vi "POC State.vi"(8 "error in (no error)":errorcluster, 11 "Node Ptr":T1 format="%.0x") -> (0 "error out":errorcluster)   [LabVIEW 2020, in "FlexRay Custom Device System Explorer.lvlib"]
uses:
  FlexRay Custom Device System Explorer.lvlib
  <vilib>/NI VeriStand/Custom Device API/Custom Device Item Ref.ctl
  <vilib>/NI VeriStand/Custom Device API/Custom Device API.lvlib
panel:
  in  "Header":cluster{"Section Name":string}={"Section Name"="Custom Device Item Settings"}
  in  "Description":string="POC State:\n0: Default Config\n1: Ready\n2: Normal Active\n3: Normal Passive\n4: Halt\n15: Config"
  in  "Name":string
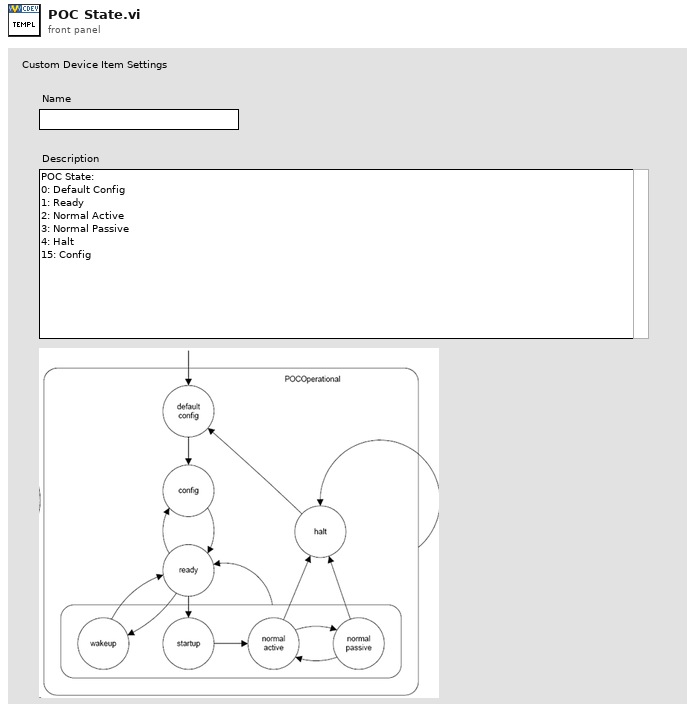
[diagram p1: front panel]
types:
  T1 = typedef "Custom Device API.lvlib/Custom Device Item Ref.ctl" = u64
  T2 = typedef "Custom Device API.lvlib/Custom Device Item Info.ctl" = cluster{"Name":string, "Is Channel":bool, "GUID":string, "Is Waveform":bool}
  T3 = typedef "Custom Device API.lvlib/Custom Device Commands.ctl" = enum16{"Default", "Item renamed", "Shutdown", "Dynamic button pressed"}
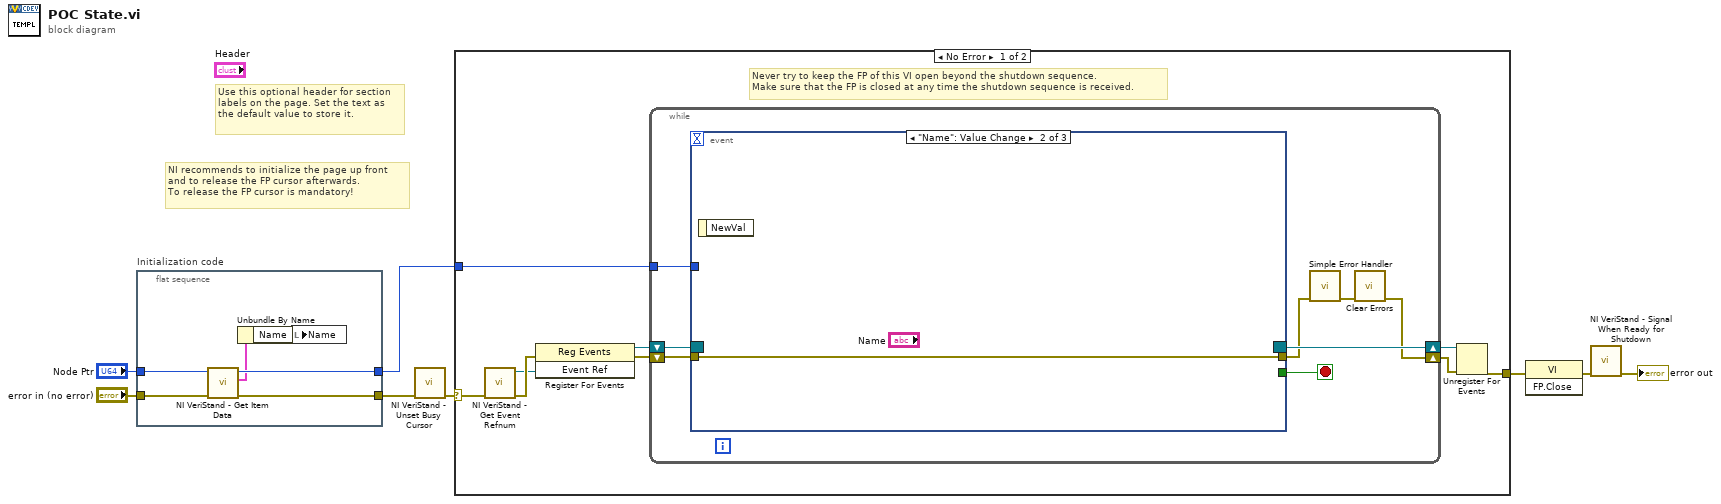
[diagram p0: block diagram]
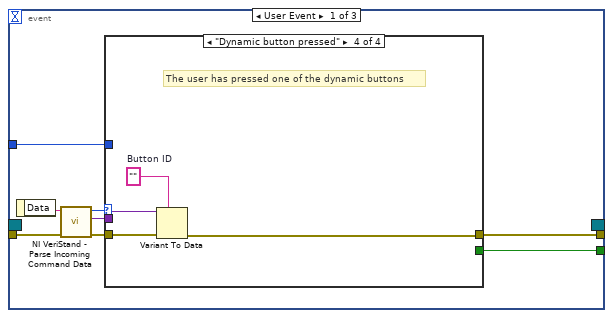
[diagram p2: hidden frame]
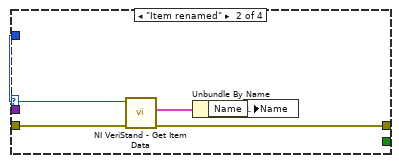
[diagram p4: hidden frame]
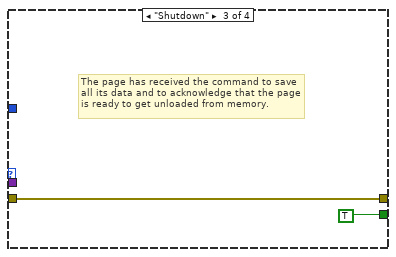
[diagram p5: hidden frame]
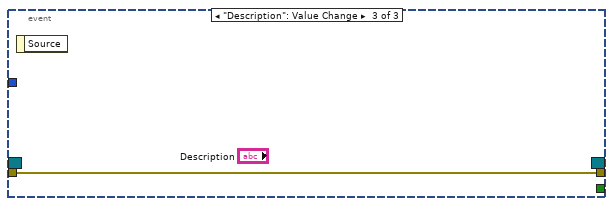
[diagram p6: hidden frame]
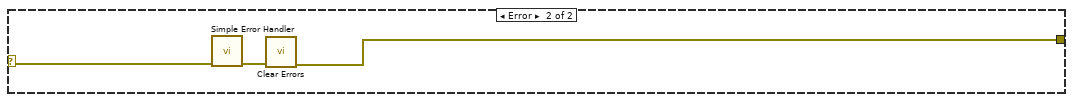
[diagram p7: hidden frame]
diagram:
  # "Use this optional header for section labels on the page. Set the text as the default value to store it."
  # "NI recommends to initialize the page up front\nand to release the FP cursor afterwards.\nTo release the FP cursor is mandatory!"
  n1 = flat-sequence "Initialization code" {
    tunnel: "error in (no error)" -> [w9]
    tunnel: "Node Ptr" -> [w10]
    tunnel: [w11] -> w4
    tunnel: [w14] -> w1
    frame #0 {
      n2 = call <vilib>:"NI VeriStand - Get Item Data.vi"("error in (no error)"=w9, "Item Ref in"=w10) -> ("error out"=w11:errorcluster, "Item Info"=w13:T2, "Item Ref out"=w14:T1)  [unwired: 7 out]
      n3 = Unbundle By Name(w13) -> ("Name"=w12:string)
      n4 = local write "Name"(w12) -> ()
    }
  }
  n5 = call <vilib>:"NI VeriStand - Unset Busy Cursor.vi"("error in (no error)"=w4) -> ("error out"=w3:errorcluster)  [unwired: 10 out]
  n6 = case shown="No Error" w3 {
    selector: w3 -> [w15 w56]
    tunnel: [w20 w54] -> w8
    tunnel: w1 -> [w16 _]
    frame No Error {
      # "Never try to keep the FP of this VI open beyond the shutdown sequence.\nMake sure that the FP is closed at any time the shutdown sequence is received."
      n7 = call <vilib>:"NI VeriStand - Get Event Refnum.vi"("error in (no error)"=w15) -> ("error out"=w23:errorcluster, "Event Ref"=w19:refnum<user-event>)  [unwired: 9 out]
      n8 = register-events(error in=w23, w19) -> (reference out=w17:refnum<event-registration>, error out=w18:errorcluster)  [unwired: 1 in]
      n9 = while {
        tunnel: w16 -> [w27]
        shift-right: [w24] -> w21
        shift-left: w18 -> [w30]
        shift-right: [w31] -> w22
        shift-left: w17 -> [w29]
        stop <- w28 stop-if-true
        n10 = event shown="[1] \"Name\": Value Change" {
          selector: w29 -> [_ _ _]
          dyn-events: [_ _ _] -> w31
          timeout: _ -> [_ _ _]
          tunnel: w30 -> [w39 w52 w53]
          tunnel: [w35 _ _] -> w28
          tunnel: [w34 w52 w53] -> w26
          tunnel: w27 -> [w33 _ _]
          event User Event {
            n11 = event-data() -> ("Data"=w38:string)  [unwired: 1 out]
            n12 = call <vilib>:"NI VeriStand - Parse Incoming Command Data.vi"("error in (no error)"=w39, "Incoming data"=w38) -> ("error out"=w37:errorcluster, "Outgoing data"=w32:variant, "Action"=w36:T3)  [unwired: 7 out]
            n13 = case shown="\"Dynamic button pressed\"" w36 {
              tunnel: w37 -> [w40 w45 w46 w51]
              tunnel: [_ _ TRUE _] -> w35
              tunnel: [w40 w42 w46 w48] -> w34
              tunnel: w33 -> [_ w44 _ _]
              tunnel: w32 -> [_ _ _ w50]
              frame "Default", Default {
              }
              frame "Item renamed" {
                n14 = call <vilib>:"NI VeriStand - Get Item Data.vi"("error in (no error)"=w45, "Item Ref in"=w44) -> ("error out"=w42:errorcluster, "Item Info"=w43:T2)  [unwired: 8 out]
                n15 = Unbundle By Name(w43) -> ("Name"=w41:string)
                n16 = local write "Name"(w41) -> ()
              }
              frame "Shutdown" {
                # "The page has received the command to save all its data and to acknowledge that the page is ready to get unloaded from memory."
              }
              frame "Dynamic button pressed" {
                w49 = ""  # Button ID
                # "The user has pressed one of the dynamic buttons"
                n17 = Variant To Data(error in=w51, type=w49, Variant=w50) -> (error out=w48:errorcluster)  [unwired: 1 out]
              }
            }
          }
          event "Name": Value Change {
            n18 = event-data() -> ()  [unwired: 2 out]
          }
          event "Description": Value Change {
            n19 = event-data() -> ()  [unwired: 2 out]
          }
        }
        n20 = call <vilib>:"Simple Error Handler.vi"("error in (no error)"=w26) -> ("error out"=w25:errorcluster)  [unwired: 1 in, 7 out]
        n21 = call <vilib>:"Clear Errors.vi"("error in (no error)"=w25) -> ("error out"=w24:errorcluster)  [unwired: 1 in, 5 out]
      }
      n22 = Unregister For Events(event registration refnum=w22, error in=w21) -> (error out=w20:errorcluster)
    }
    frame Error {
      n23 = call <vilib>:"Simple Error Handler.vi"("error in (no error)"=w56) -> ("error out"=w55:errorcluster)  [unwired: 1 in, 7 out]
      n24 = call <vilib>:"Clear Errors.vi"("error in (no error)"=w55) -> ("error out"=w54:errorcluster)  [unwired: 1 in, 5 out]
    }
  }
  n25 = invoke class="VI" method="FP.Close"(error in=w8) -> (error out=w7:errorcluster)  [unwired: 2 in, 2 out]
  n26 = call <vilib>:"NI VeriStand - Signal When Ready for Shutdown.vi"("error in (no error)"=w7) -> ("error out"=→"error out":errorcluster)  [unwired: 10 out]
